vi "PCO_RecorderGetStatus.vi"(0 "phRec":u64, 1 "phCam":u64, 5 "error in (no error)":errorcluster {"code" format="%x"}) -> (6 "dwStartTime":u32, 7 "dwStopTime":u32, 10 "bBuffersFull":bool, 11 "bFIFOOverflow":bool, 12 "dwProcImgCount":u32, 13 "dwReqImgCount":u32, 14 "phRec out":u64, 15 "ErrorMessage":i32 format="%x", 16 "bIsRunning":bool, 17 "bAutoExpState":bool, 18 "dwLastError":u32 format="%x", 19 "error out":errorcluster {"code" format="%x"})   [LabVIEW 2019, in "Recorder.lvlib"]
doc: "<b>Description:</b>\nThis function retrieves the current recorder status for a specific camera.\n\n<b>Supported camera type:</b>\nAll cameras"
uses:
  Recorder.lvlib
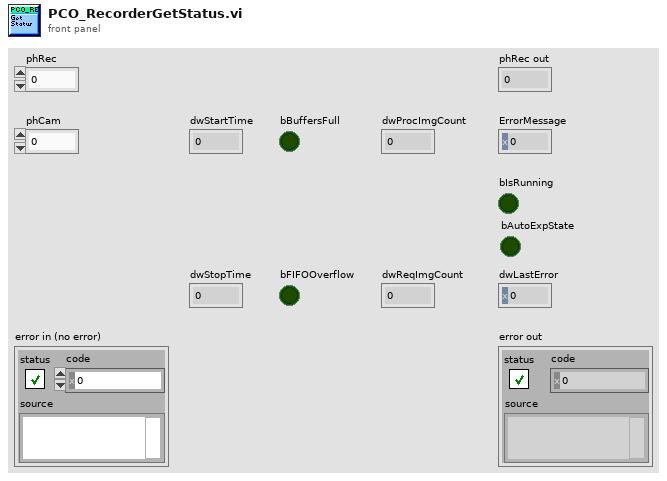
[diagram p1: front panel]
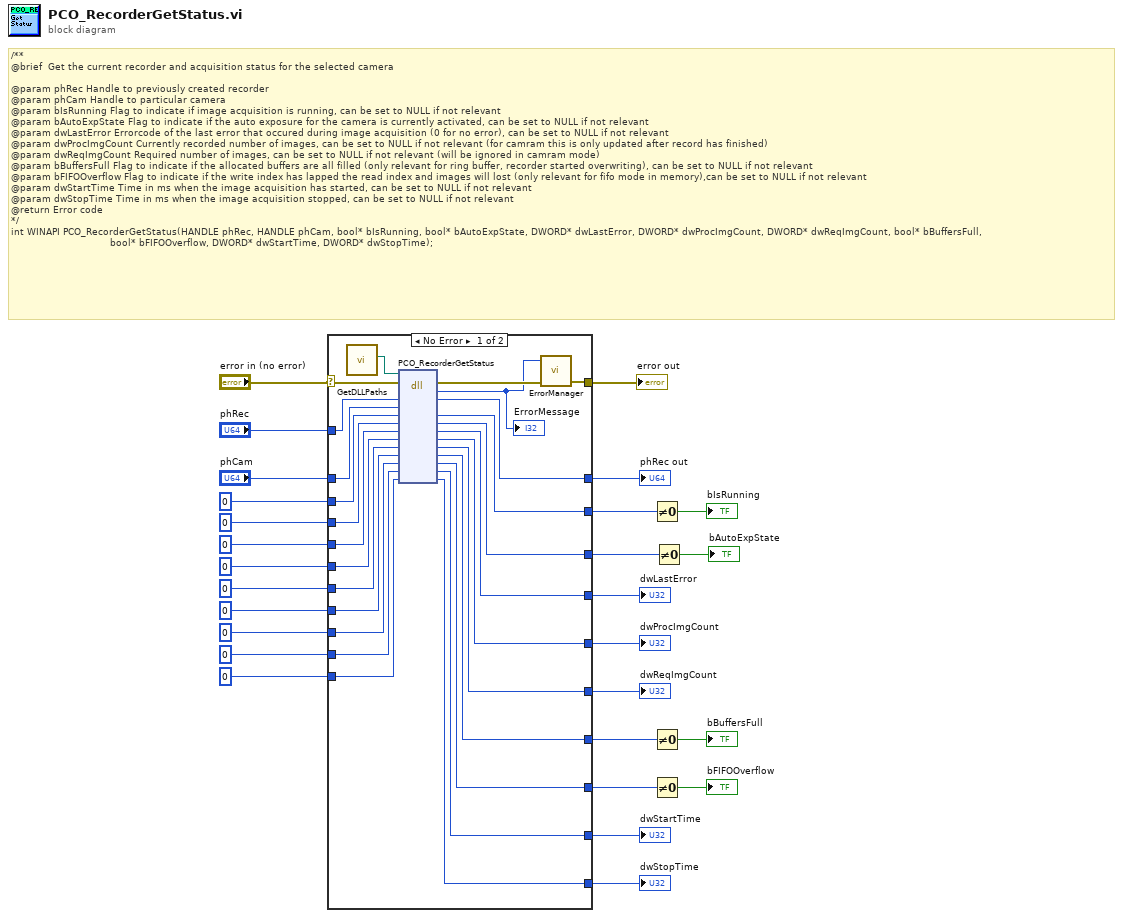
[diagram p0: block diagram]
diagram:
  # "/**\n@brief \tGet the current recorder and acquisition status for the selected camera\n\n@param phRec Handle to previously created recorder\n@param phCam Handle to particular camera\n@param bIsRunning Flag to indicate if image acquisition is running, can be set to NULL if not relevant\n@param bAutoExpState Flag to indicate if the auto exposure for the camera is currently activated, can be set to NULL if not relevant\n@param dwLastError Errorcode of the last error that occured during image acquisition (0 for no error), can be set to NULL if not relevant\n@param dwProcImgCount Currently recorded number of images, can be set to NULL if not relevant (for camram this is only updated after record has finished)\n@param dwReqImgCount Required number of images, can be set to NULL if not relevant (will be ignored in camram mode)\n@param bBuffersFull Flag to indicate if the allocated buffers are all filled (only relevant for ring buffer, recorder started overwriting), can be set to NULL if not relevant\n@param bFIFOOverflow Flag to indicate if the write index has lapped the read index and images will lost (only relevant for fifo mode in memory),can be set to NULL if not relevant\n@param dwStartTime Time in ms when the image acquisition has started, can be set to NULL if not relevant\n@param dwStopTime Time in ms when the image acquisition stopped, can be set to NULL if not relevant\n@return Error code\n*/\nint WINAPI PCO_RecorderGetStatus(HANDLE phRec, HANDLE phCam, bool* bIsRunning, bool* bAutoExpState, DWORD* dwLastError, DWORD* dwProcImgCount, DWORD* dwReqImgCount, bool* bBuffersFull,\n                                 bool* bFIFOOverflow, DWORD* dwStartTime, DWORD* dwStopTime);"
  n1 = case shown="No Error" "error in (no error)" {
    selector: "error in (no error)" -> [w34 w64]
    tunnel: "phRec" -> [w53 w63]
    tunnel: [w52 w63] -> w26
    tunnel: "phCam" -> [w51 _]
    tunnel: u8 0 ("bIsRunning") -> [w50 w62]
    tunnel: [w49 w62] -> w22
    tunnel: u32 0 ("dwLastError") -> [w48 w61]
    tunnel: [w47 w61] -> w20
    tunnel: u32 0 ("dwProcImgCount") -> [w46 w60]
    tunnel: [w45 w60] -> w18
    tunnel: u32 0 ("dwReqImgCount") -> [w44 w59]
    tunnel: [w43 w59] -> w16
    tunnel: u8 0 ("bBuffersFull") -> [w42 w58]
    tunnel: [w41 w58] -> w13
    tunnel: u8 0 ("bFIFOOverflow") -> [w40 w57]
    tunnel: [w39 w57] -> w10
    tunnel: u32 0 ("dwStartTime") -> [w38 w56]
    tunnel: [w37 w56] -> w8
    tunnel: u32 0 ("dwStopTime") -> [w36 w55]
    tunnel: [w35 w55] -> w6
    tunnel: [w33 w64] -> w5
    tunnel: u32 0 ("dwLastError") -> [w30 w54]
    tunnel: [w29 w54] -> w1
    frame No Error {
      n2 = call "GetDLLPaths.vi"() -> ("PCO_Recorder_Path"=w28:path)  [unwired: 8 in, 3 out]
      n3 = dll-call lib="?" fn="PCO_RecorderGetStatus"(path in=w28, error in=w34, "phRec"=w53, "phCam"=w51, "bIsRunning"=w50, "bAutoExpState"=w30, "dwLastError"=w48, "dwProcImgCount"=w46, "dwReqImgCount"=w44, "bBuffersFull"=w42, "bFIFOOverflow"=w40, "dwStartTime"=w38, "dwStopTime"=w36) -> (error out=w32:errorcluster, "return type"=w31:i32, "phRec"=w52:u64, "bIsRunning"=w49:u8, "bAutoExpState"=w29:u8, "dwLastError"=w47:u32, "dwProcImgCount"=w45:u32, "dwReqImgCount"=w43:u32, "bBuffersFull"=w41:u8, "bFIFOOverflow"=w39:u8, "dwStartTime"=w37:u32, "dwStopTime"=w35:u32)  [unwired: 2 in, 1 out]
      "ErrorMessage" <- w31
      n4 = call "ErrorManager.vi"("error in (no error)"=w32, "error code"=w31) -> ("error out"=w33:errorcluster)  [unwired: 2 in, 1 out]
    }
    frame Error {
    }
  }
  "phRec out" <- w26
  "dwLastError" <- w20
  "dwProcImgCount" <- w18
  "dwReqImgCount" <- w16
  "dwStartTime" <- w8
  "dwStopTime" <- w6
  "error out" <- w5
  n5 = Not Equal To 0?(x=w22) -> (x != 0?=→"bIsRunning":bool)
  n6 = Not Equal To 0?(x=w13) -> (x != 0?=→"bBuffersFull":bool)
  n7 = Not Equal To 0?(x=w10) -> (x != 0?=→"bFIFOOverflow":bool)
  n8 = Not Equal To 0?(x=w1) -> (x != 0?=→"bAutoExpState":bool)
